vi "BASE_I_O_Manual.vi"(8 "error in (no error)":errorcluster) -> (0 "error out":errorcluster)   [LabVIEW 2017]
doc: "This vi is for manually turn ON and OFF also monitor Output of PLCS. So this is manual screen."
uses:
  Global/PLC_to_Auto.vi
  <vilib>/Utility/file.llb/Read Delimited Spreadsheet (string).vi
panel:
  out "SAMPLE":bool
  out "X27-SPARE 2":bool
  out "X26-SPARE 2":bool
  out "X26-SPARE":bool
  out "X25-REJECTION FULL SENSOR":bool
  out "X24-REJECTION SENSOR":bool
  out "X23-DOOR 4":bool
  out "X22-DOOR 3":bool
  out "X27-SPARE":bool
  out "PART CLAMP END RS":bool
  out "UP DOWN CYL END RS":bool
  out "UP DOWN CYL  HM RS":bool
  out "PUSHER END RS":bool
  out "PUSHER HM RS":bool
  out "THREAD LOCKER CYL COMPLETE":bool
  out "SHUTTLE OPEN CHECK SENSOR-X300":bool
  out "SPARE":bool
  out "DOOR 2":bool
  out "DOOR 1":bool
  out "SAFETY SENSOR":bool
  out "PRESSURE SWITCH":bool
  out "RESET PB":bool
  out "EMG STOP":bool
  out "CYCLE START TOUCH BUTTON 2":bool
  out "CYCLE START TOUCH BUTTON 1":bool
  in  "Tab Control":enum32{"MANUAL CYCLE"}(tab)
  in  "Cluster - Thin Border":T1
  in  "Back":bool
  # "Manual Cycle"
  # "INPUT"
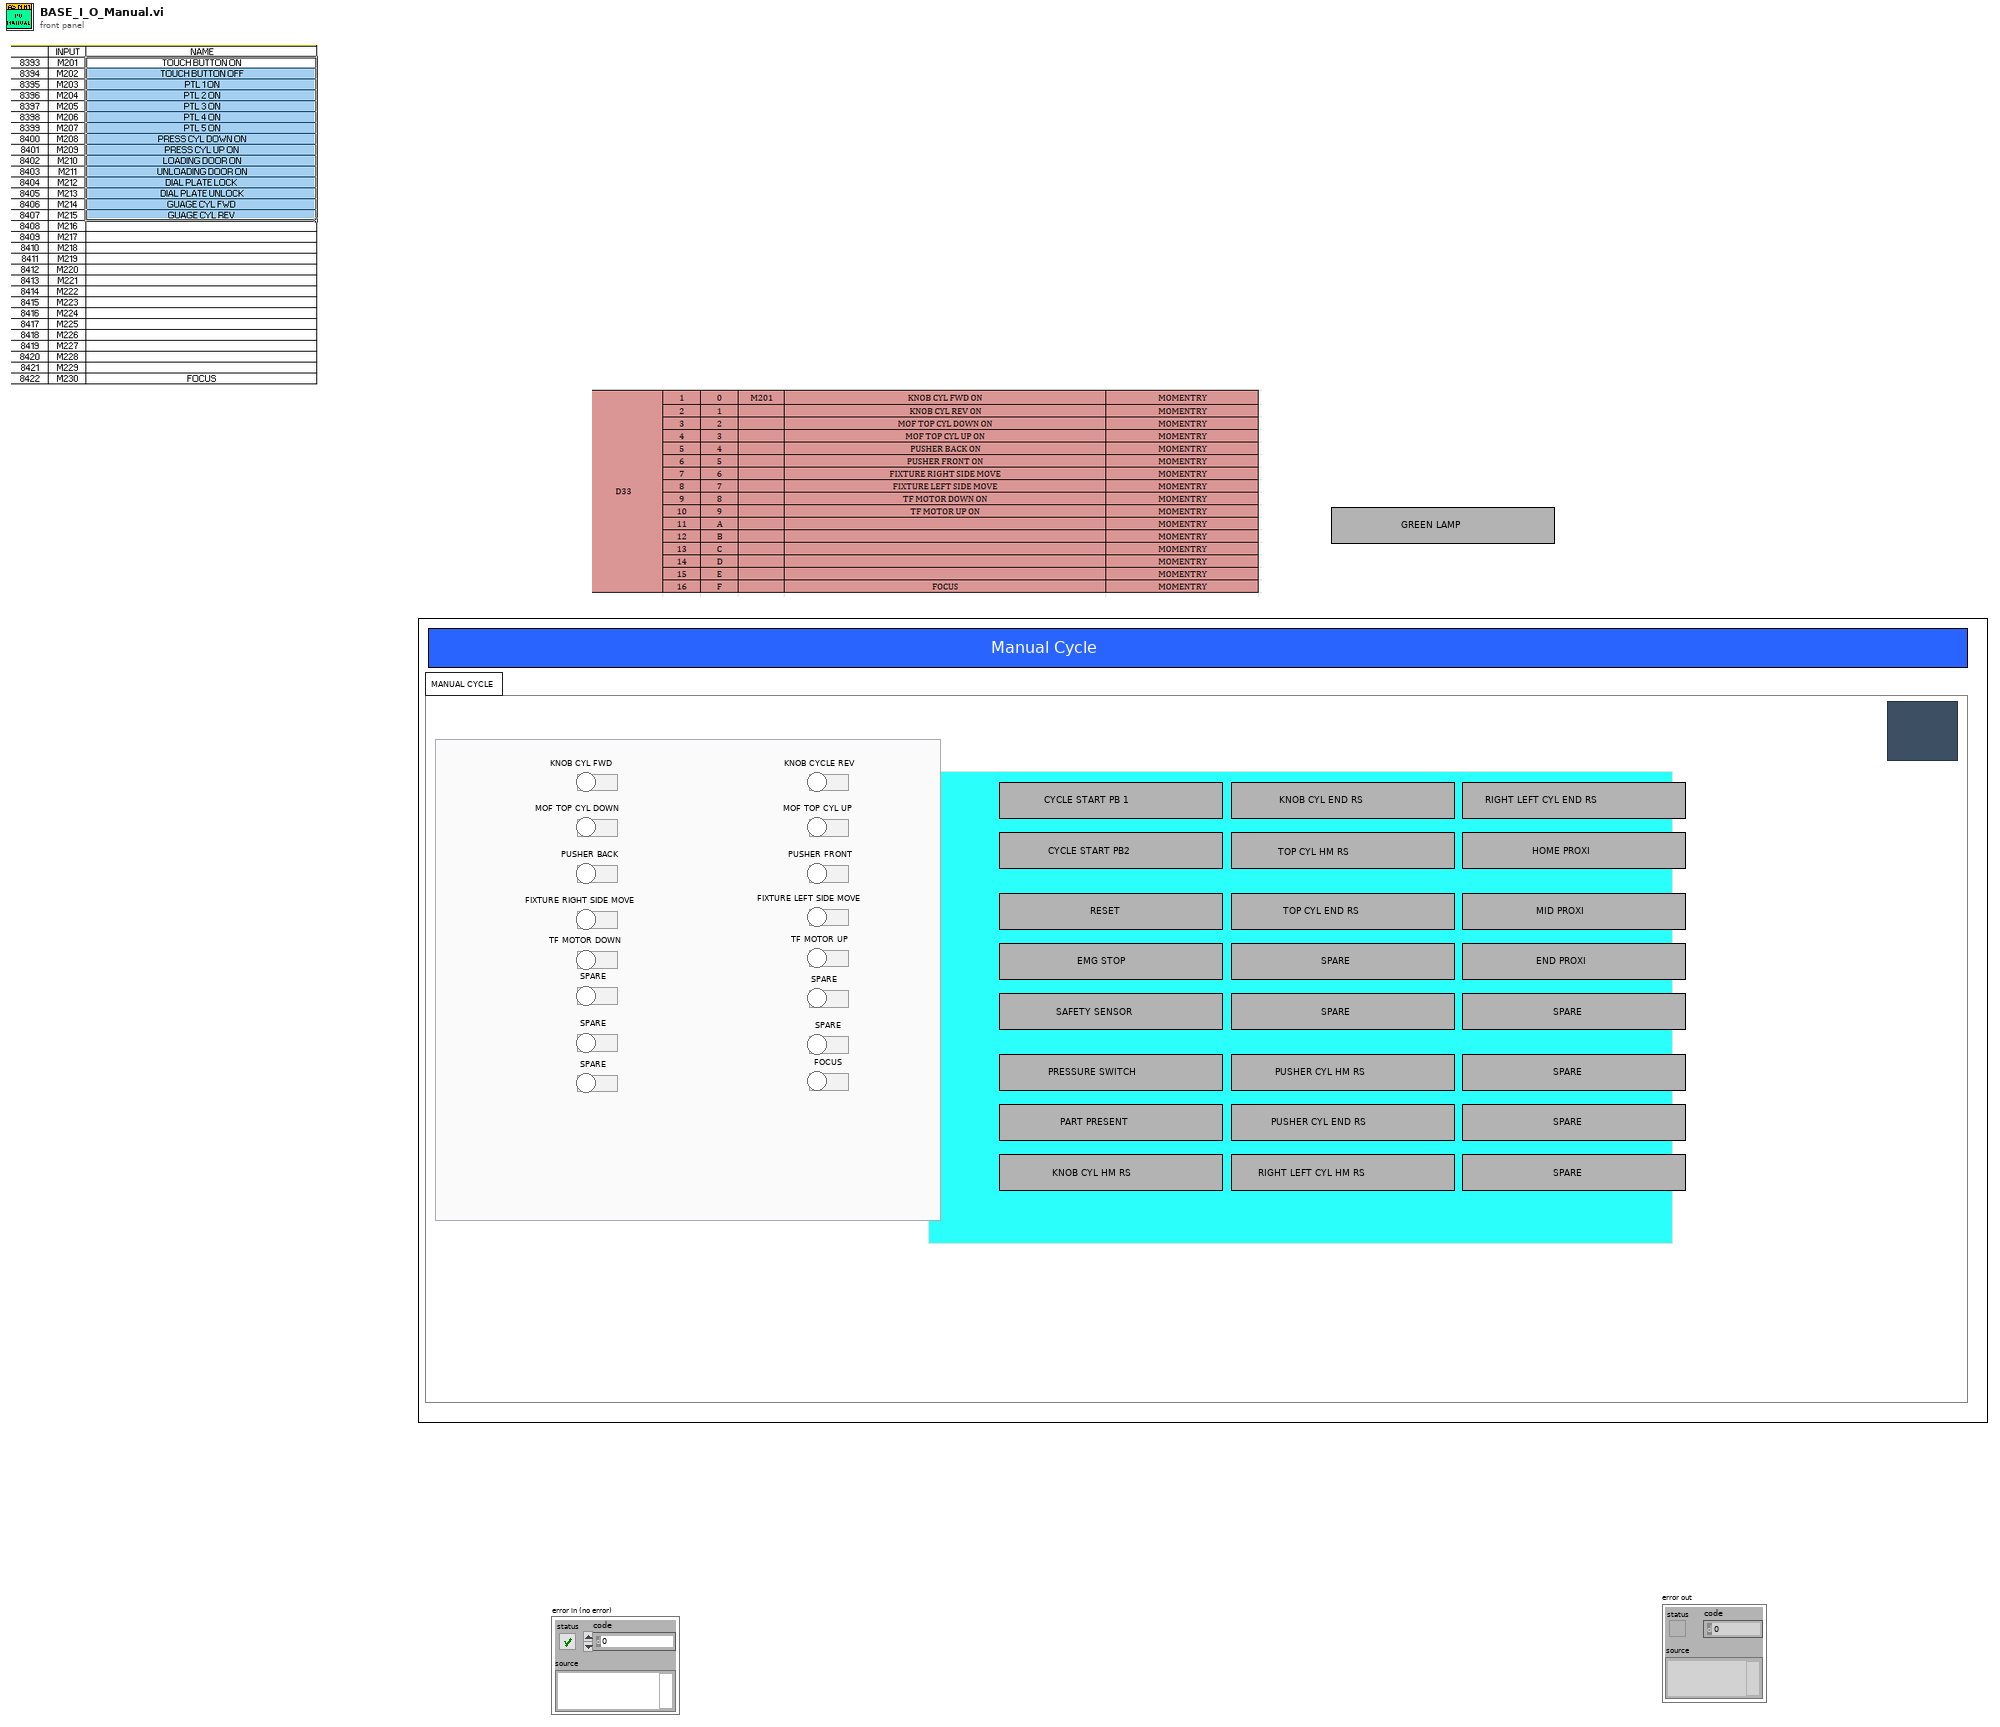
[diagram p1: front panel]
types:
  T1 = cluster{"KNOB CYL FWD":bool, "KNOB CYCLE REV":bool, "MOF TOP CYL DOWN":bool, "MOF TOP CYL UP":bool, "PUSHER BACK":bool, "PUSHER FRONT":bool, "FIXTURE RIGHT SIDE MOVE":bool, "FIXTURE LEFT SIDE MOVE":bool, "TF MOTOR DOWN":bool, "TF MOTOR UP":bool, "SPARE":bool, "SPARE":bool, "SPARE":bool, "SPARE":bool, "SPARE":bool, "FOCUS":bool}
  T2 = enum32{"invalid app kind", "Development System", "Run Time System", "Student Edition", "Embedded LabVIEW", "Evaluation", "Custom"}
  T3 = enum32{"Invalid", "Standard", "Closed", "Hidden", "Minimized", "Maximized"}
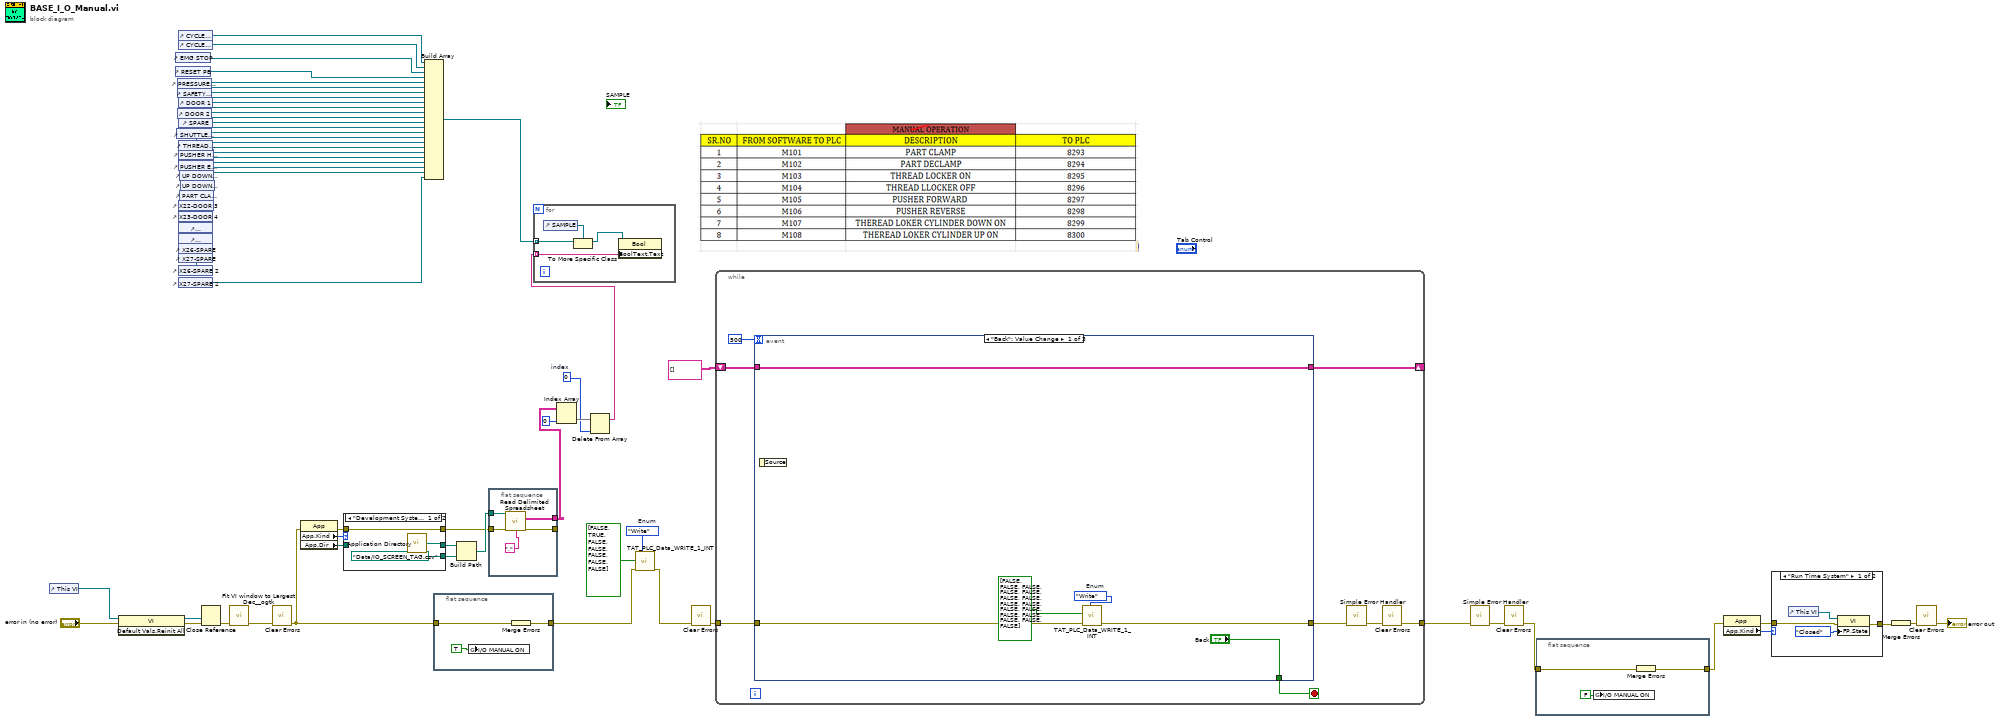
[diagram p0: block diagram]
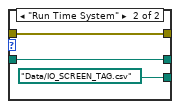
[diagram p2: hidden frame]
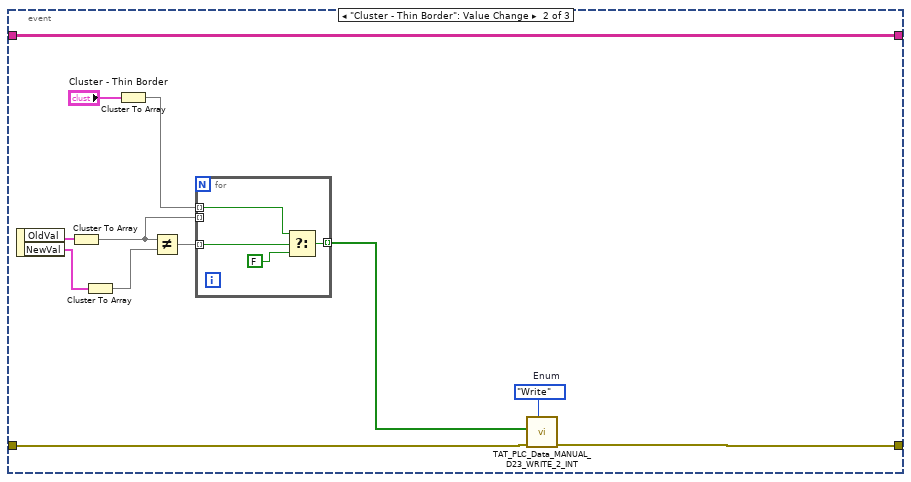
[diagram p4: hidden frame]
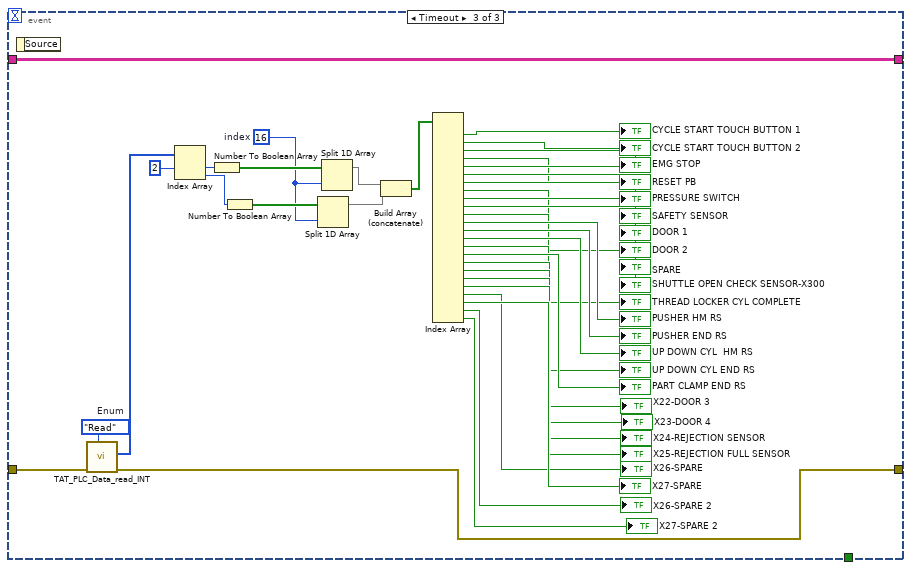
[diagram p5: hidden frame]
diagram:
  w9 = enum16{"Read", "Write"}."Write"  # Enum
  w40 = 0  # index
  n1 = control-ref of="This VI"() -> (w54:refnum<vi>)
  n2 = invoke class="VI" method="Default Vals.Reinit All"(reference=w54, error in="error in (no error)") -> (reference out=w52:refnum<vi>, error out=w51:errorcluster)  [unwired: 1 in, 1 out]
  n3 = control-ref of="EMG STOP"() -> (w3:refnum<vi>)
  n4 = control-ref of="RESET PB"() -> (w31:refnum<vi>)
  n5 = control-ref of="SHUTTLE OPEN CHECK SENSOR-X300"() -> (w25:refnum<vi>)
  n6 = control-ref of="PRESSURE SWITCH"() -> (w30:refnum<vi>)
  n7 = control-ref of="SAFETY SENSOR"() -> (w29:refnum<vi>)
  n8 = control-ref of="DOOR 2"() -> (w27:refnum<vi>)
  n9 = control-ref of="CYCLE START TOUCH BUTTON 1"() -> (w5:refnum<vi>)
  n10 = control-ref of="CYCLE START TOUCH BUTTON 2"() -> (w4:refnum<vi>)
  n11 = control-ref of="DOOR 1"() -> (w28:refnum<vi>)
  n12 = control-ref of="SPARE"() -> (w26:refnum<vi>)
  n13 = control-ref of="THREAD LOCKER CYL COMPLETE"() -> (w24:refnum<vi>)
  n14 = control-ref of="X23-DOOR 4"() -> (w17:refnum<vi>)
  n15 = control-ref of="X24-REJECTION SENSOR"() -> (w16:refnum<vi>)
  n16 = control-ref of="X25-REJECTION FULL SENSOR"() -> (w15:refnum<vi>)
  n17 = control-ref of="X26-SPARE"() -> (w14:refnum<vi>)
  n18 = control-ref of="X27-SPARE"() -> (w13:refnum<vi>)
  n19 = control-ref of="X26-SPARE 2"() -> (w12:refnum<vi>)
  n20 = control-ref of="X27-SPARE 2"() -> (w11:refnum<vi>)
  n21 = control-ref of="PUSHER HM RS"() -> (w23:refnum<vi>)
  n22 = control-ref of="PUSHER END RS"() -> (w22:refnum<vi>)
  n23 = control-ref of="X22-DOOR 3"() -> (w18:refnum<vi>)
  n24 = control-ref of="UP DOWN CYL  HM RS"() -> (w21:refnum<vi>)
  n25 = control-ref of="PART CLAMP END RS"() -> (w19:refnum<vi>)
  n26 = control-ref of="UP DOWN CYL END RS"() -> (w20:refnum<vi>)
  n27 = Close Reference(reference=w52, error in (no error)=w51) -> (error out=w50:errorcluster)
  n28 = call <userlib>:"Fit VI window to Largest Dec__ogtk.vi"("error in (no error)"=w50) -> ("error out"=w44:errorcluster)  [unwired: 5 in, 1 out]
  n29 = call <vilib>:"Clear Errors.vi"("error in (no error)"=w44) -> ("error out"=w2:errorcluster)  [unwired: 5 in, 1 out]
  n30 = property class="App"(error in=w2) -> (error out=w38:errorcluster, "App.Kind"=w34:T2, "App.Dir"=w35:path)  [unwired: 1 in, 1 out]
  n31 = case shown="\"Development System\", Default" w34 {
    tunnel: [w62 w65] -> w1
    tunnel: w38 -> [w62 w65]
    tunnel: w35 -> [_ w64]
    tunnel: [w60 w64] -> w37
    tunnel: [path "Data/IO_SCREEN_TAG.csv" path "Data/IO_SCREEN_TAG.csv"] -> w36
    frame "Development System", Default {
      n32 = call <vilib>:"Application Directory.vi"() -> ("Application Directory"=w60:path)
    }
    frame "Run Time System" {
    }
  }
  n33 = Build Array(w5, w4, w3, w31, w30, w29, w28, w27, w26, w25, w24, w23, w22, w21, w20, w19, w18, w17, w16, w15, w14, w13, w12, w11) -> (w39:refnum<vi>[])
  n34 = flat-sequence {
    tunnel: w2 -> [w68]
    tunnel: [w67] -> w7
    frame #0 {
      n35 = global write "PLC_to_Auto.vi" "I/O MANUAL ON"(TRUE) -> ()
      n36 = Merge Errors(w68) -> (w67:errorcluster)
    }
  }
  n37 = Build Path(base path=w37, name or relative path=w36) -> (appended path=w33:path)
  n38 = flat-sequence {
    tunnel: w1 -> [w72]
    tunnel: [w73] -> _
    tunnel: w33 -> [w71]
    tunnel: [w69] -> w32
    frame #0 {
      n39 = call-poly <vilib>:"Read Delimited Spreadsheet.vi"("file path (dialog if empty)"=w71, "error in (no error)"=w72, "delimiter (\\t)"=",") -> ("all rows"=w69:string[][], "error out"=w73:errorcluster)  [unwired: 7 in, 4 out]
    }
  }
  n40 = Index Array(array=w32, index (col)=0) -> (element=w41:string[])  [unwired: 1 in]
  n41 = Delete From Array(array=w41, index=w40) -> (array with subset deleted=w10:string[])  [unwired: 1 in, 1 out]
  n42 = for {
    tunnel: w10 -> [w76] mode=indexing
    tunnel: w39 -> [w75] mode=indexing
    n43 = control-ref of="SAMPLE"() -> (w74:refnum<vi>)
    n44 = To More Specific Class(target class=w74, reference=w75) -> (specific class reference=w77:refnum<vi>)  [unwired: 1 in, 1 out]
    n45 = property on="Property Node" class="Bool"(reference=w77, "BoolText.Text"=w76) -> ()  [unwired: 1 in, 2 out]
  }
  n46 = call "TAT_PLC_Data_WRITE_1_INT.vi"("Enum"=w9, "error in (no error)"=w7, "Array"=bool[] [FALSE, TRUE, FALSE, FALSE, FALSE, FALSE, FALSE]) -> ("error out"=w6:errorcluster)  [unwired: 7 in, 1 out]
  n47 = call <vilib>:"Clear Errors.vi"("error in (no error)"=w6) -> ("error out"=w43:errorcluster)  [unwired: 5 in, 1 out]
  n48 = while {
    tunnel: w43 -> [w85]
    tunnel: [w78] -> w58
    shift-right: [w83] -> _
    shift-left: string[][] [] -> [w82]
    stop <- w84 stop-if-true
    n49 = event shown="[0] \"Back\": Value Change" {
      selector: _ -> [_ _ _]
      dyn-events: _ -> [_ _ _]
      timeout: 500 -> [_ _ _]
      tunnel: w85 -> [w88 w96 w109]
      tunnel: [w87 w95 w108] -> w80
      tunnel: ["Back" _ _] -> w84
      tunnel: [w90 w103 w145] -> w83
      tunnel: w82 -> [w90 w103 w145]
      event "Back": Value Change {
        w89 = enum16{"Read", "Write"}."Write"  # Enum
        n50 = event-data() -> ()  [unwired: 1 in, 1 out]
        n51 = call "TAT_PLC_Data_WRITE_1_INT.vi"("Enum"=w89, "error in (no error)"=w88, "Array"=bool[] [FALSE, FALSE, FALSE, FALSE, FALSE, FALSE, FALSE, FALSE, FALSE, FALSE, FALSE, FALSE, FALSE, FALSE, FALSE, FALSE]) -> ("error out"=w87:errorcluster)  [unwired: 7 in, 1 out]
      }
      event "Cluster - Thin Border": Value Change {
        w94 = enum16{"Read", "Write"}."Write"  # Enum
        n52 = event-data() -> ("OldVal"=w101:T1, "NewVal"=w100:T1)  [unwired: 1 in]
        n53 = Cluster To Array(cluster=w101) -> (array=w98:bool[])
        n54 = Cluster To Array(cluster=w100) -> (array=w99:bool[])
        n55 = Cluster To Array(cluster="Cluster - Thin Border") -> (array=w93:bool[])
        n56 = Not Equal?(x=w98, y=w99) -> (x != y?=w97:bool[])
        n57 = for {
          tunnel: w93 -> [w106] mode=indexing
          tunnel: w98 -> [_] mode=indexing
          tunnel: w97 -> [w107] mode=indexing
          tunnel: [w105] -> w92 mode=indexing
          n58 = Select(t=w106, s=w107, f=FALSE) -> (s? t:f=w105:bool)
        }
        n59 = call "TAT_PLC_Data_MANUAL_D23_WRITE_2_INT.vi"("Enum"=w94, "error in (no error)"=w96, "Array"=w92) -> ("error out"=w95:errorcluster)  [unwired: 7 in, 1 out]
      }
      event Timeout {
        w112 = 16  # index
        w110 = enum16{"Read", "Write"}."Read"  # Enum
        n60 = event-data() -> ()  [unwired: 1 in, 1 out]
        n61 = call "TAT_PLC_Data_read_INT.vi"("Enum"=w110, "error in (no error)"=w109) -> ("error out"=w108:errorcluster, "Array 2"=w137:u16[])  [unwired: 8 in]
        n62 = Index Array(array=w137, index #1=2) -> (element #1=w138:u16, element #2=w141:u16)  [unwired: 1 in]
        n63 = Number To Boolean Array(number=w138) -> (Boolean array=w139:bool[])
        n64 = Number To Boolean Array(number=w141) -> (Boolean array=w140:bool[])
        n65 = Split 1D Array(array=w140, index=w112) -> (first subarray=w144:bool[])  [unwired: 1 out]
        n66 = Split 1D Array(array=w139, index=w112) -> (first subarray=w142:bool[])  [unwired: 1 out]
        n67 = Build Array (concatenate)(w142, w144) -> (w143:bool[])
        n68 = Index Array(array=w143) -> (element #1=→"CYCLE START TOUCH BUTTON 1":bool, element #2=→"CYCLE START TOUCH BUTTON 2":bool, element #3=→"EMG STOP":bool, element #4=→"RESET PB":bool, element #5=→"PRESSURE SWITCH":bool, element #6=→"SAFETY SENSOR":bool, element #7=→"DOOR 1":bool, element #8=→"DOOR 2":bool, element #9=→"SPARE":bool, element #10=→"SHUTTLE OPEN CHECK SENSOR-X300":bool, element #11=→"THREAD LOCKER CYL COMPLETE":bool, element #12=→"PUSHER HM RS":bool, element #13=→"PUSHER END RS":bool, element #14=→"UP DOWN CYL  HM RS":bool, element #15=→"UP DOWN CYL END RS":bool, element #16=→"PART CLAMP END RS":bool, element #17=→"X22-DOOR 3":bool, element #18=→"X23-DOOR 4":bool, element #19=→"X24-REJECTION SENSOR":bool, element #20=→"X25-REJECTION FULL SENSOR":bool, element #21=→"X26-SPARE":bool, element #22=→"X27-SPARE":bool, element #23=→"X26-SPARE 2":bool, element #24=→"X27-SPARE 2":bool)  [unwired: 24 in]
      }
    }
    n69 = call <vilib>:"Simple Error Handler.vi"("error in (no error)"=w80) -> ("error out"=w79:errorcluster)  [unwired: 4 in, 4 out]
    n70 = call <vilib>:"Clear Errors.vi"("error in (no error)"=w79) -> ("error out"=w78:errorcluster)  [unwired: 5 in, 1 out]
  }
  n71 = call <vilib>:"Simple Error Handler.vi"("error in (no error)"=w58) -> ("error out"=w49:errorcluster)  [unwired: 4 in, 4 out]
  n72 = call <vilib>:"Clear Errors.vi"("error in (no error)"=w49) -> ("error out"=w46:errorcluster)  [unwired: 5 in, 1 out]
  n73 = flat-sequence {
    tunnel: w46 -> [w148]
    tunnel: [w147] -> w45
    frame #0 {
      n74 = global write "PLC_to_Auto.vi" "I/O MANUAL ON"(FALSE) -> ()
      n75 = Merge Errors(w148) -> (w147:errorcluster)
    }
  }
  n76 = property class="App"(error in=w45) -> (error out=w47:errorcluster, "App.Kind"=w48:T2)  [unwired: 1 in, 1 out]
  n77 = case shown="\"Run Time System\"" w48 {
    tunnel: w47 -> [w150 w153]
    tunnel: [w149 w153] -> w56
    frame "Run Time System" {
      n78 = control-ref of="This VI"() -> (w152:refnum<vi>)
      n79 = property class="VI"(reference=w152, error in=w150, "FP.State"=T3."Closed" ("Front Panel Window:State")) -> (error out=w149:errorcluster)  [unwired: 1 out]
    }
    frame "Development System", Default {
    }
  }
  n80 = Merge Errors(w56) -> (w57:errorcluster)
  n81 = call <vilib>:"Clear Errors.vi"("error in (no error)"=w57) -> ("error out"=→"error out":errorcluster)  [unwired: 5 in, 1 out]
